vi "ByViServerInterfaceTemplate_6x8x6_Method.vi"(0 "Interface In(KEEP)":refnum<class>, 5 "error in (no error)":errorcluster) -> (14 "Interface Out(KEEP)":refnum<class>, 19 "error out":errorcluster)   [LabVIEW 2012]
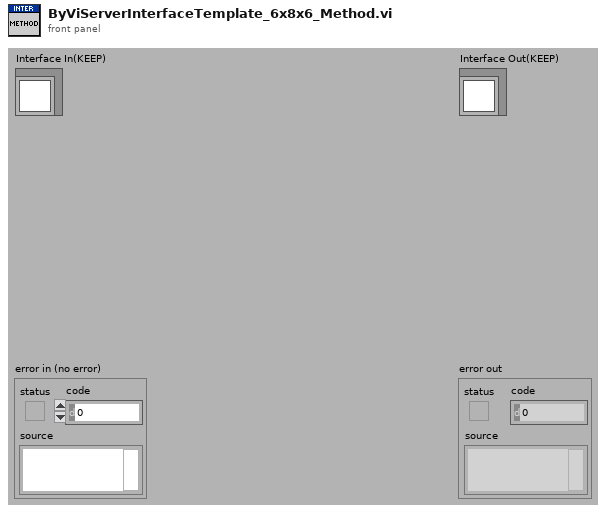
[diagram p1: front panel]
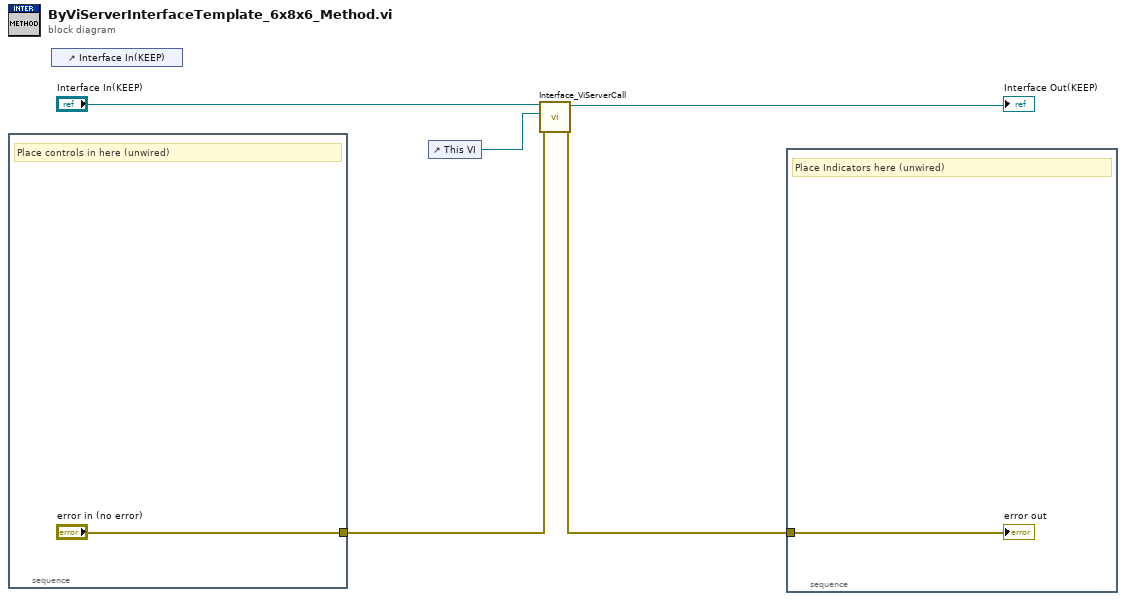
[diagram p0: block diagram]
diagram:
  n1 = stacked-sequence {
    tunnel: ["error in (no error)"] -> w3
    frame #0 {
      # "Place controls in here (unwired)"
    }
  }
  n2 = control-ref of="Interface In(KEEP)"() -> ()  [unwired: 1 out]
  n3 = control-ref of="This VI"() -> (w1:refnum<vi>)
  n4 = call <vilib>:"Interface_ViServerCall.vi"("error in (no error)"=w3, "This VI"=w1, "LabVIEW Object in"="Interface In(KEEP)") -> ("error out"=w2:errorcluster, "LabVIEW Object out"=→"Interface Out(KEEP)":refnum<class>)  [unwired: 7 in]
  n5 = stacked-sequence {
    tunnel: w2 -> [w7]
    frame #0 {
      # "Place Indicators here (unwired)"
      "error out" <- w7
    }
  }
